vi "TDMS Write.vi"(7 "Channel Name":string, 8 "error in (no error)":errorcluster, 9 "Group Name":string, 10 "TDMS in":refnum<k34>, 11 "Enum Array in":refnum<class "Enum Array.lvclass">) -> (0 "error out":errorcluster, 2 "TDMS Out":refnum<k34>)   [LabVIEW 2020, in "Data.lvlib" / "Enum Array.lvclass"]
doc: "Write Generic Data to a TDMS file.\nThis implementation writes the Enum index with 'Channel Name' and the Enum Alias as 'Channel Name'_Alias."
uses:
  Enum Array.lvclass
  Enum Array.lvclass/Enum Array.ctl
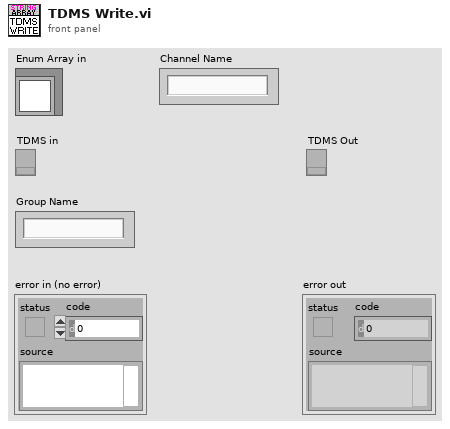
[diagram p1: front panel]
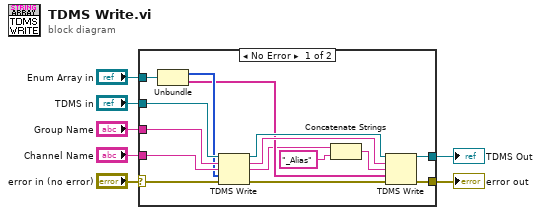
[diagram p0: block diagram]
diagram:
  n1 = case shown="No Error" "error in (no error)" {
    selector: "error in (no error)" -> [w22 w23]
    tunnel: [w15 w23] -> w6
    tunnel: "TDMS in" -> [w20 w24]
    tunnel: [w13 w24] -> w5
    tunnel: "Channel Name" -> [w19 _]
    tunnel: "Group Name" -> [w18 _]
    tunnel: "Enum Array in" -> [w17 _]
    frame No Error {
      n2 = Unbundle(w17) -> (w16:u32[], w11:string[])
      n3 = TDMS Write(0:w20, 5:w18, 7:w19, 9:w16, 11:w22) -> (4:w14:refnum<k34>, 6:w12:string, 8:w9:string, 15:w21:errorcluster)  [unwired: 1 in]
      n4 = Concatenate Strings(w9, "_Alias" ("string")) -> (w8:string)
      n5 = TDMS Write(0:w14, 5:w12, 7:w8, 9:w11, 11:w21) -> (4:w13:refnum<k34>, 15:w15:errorcluster)  [unwired: 1 in, 2 out]
    }
    frame Error {
    }
  }
  "error out" <- w6
  "TDMS Out" <- w5
